vi "output.vi"(8 "error in":errorcluster, 10 "data table in":T1, 11 "SystemLin Tag Module runtime in":refnum<class "SystemLink File runtime.lvclass">) -> (0 "error out":errorcluster, 2 "data table out":T1, 3 "SystemLin Tag Module runtime out":refnum<class "SystemLink File runtime.lvclass">)   [LabVIEW 2015, in "SystemLink File runtime.lvclass"]
doc: "Provides an interface for writing data to a module at runtime. While this interface performs no operations, a child should provide an override which may write to any open sessions, references, or interfaces."
uses:
  SystemLink File runtime.lvclass
  <vilib>/NI/Tag Bus/table/data table.ctl
  SystemLink File runtime.lvclass/SystemLink File runtime.ctl
  <vilib>/NI/Tag Bus/table/data polymorphs/read one/read Boolean.vi
  <vilib>/Skyline/File/File/Send File.vi
  <vilib>/NI/Tag Bus/table/data table.lvlib
  <vilib>/NI/Tag Bus/table/data polymorphs/read one/read Double.vi
  <vilib>/NI/Tag Bus/table/data polymorphs/read one/read Single.vi
  <vilib>/NI/Tag Bus/table/data polymorphs/read one/read I32.vi
  <vilib>/NI/Tag Bus/table/data polymorphs/read one/read I16.vi
  <vilib>/NI/Tag Bus/table/data polymorphs/read one/read I8.vi
  <vilib>/Skyline/Tag/Wrapper/Wrapper_class/NI Skyline Tag.lvclass
  <vilib>/Skyline/Tag/Wrapper/Wrapper_class/Write Tag (DBL).vi
  <vilib>/Skyline/Tag/Wrapper/Wrapper_class/Write Tag (I32).vi
  <vilib>/NI/Tag Bus/table/data polymorphs/read one/read String.vi
  <vilib>/Skyline/Tag/Wrapper/Wrapper_class/Write Tag (String).vi
  <vilib>/Skyline/File/File/NI Skyline File.lvclass
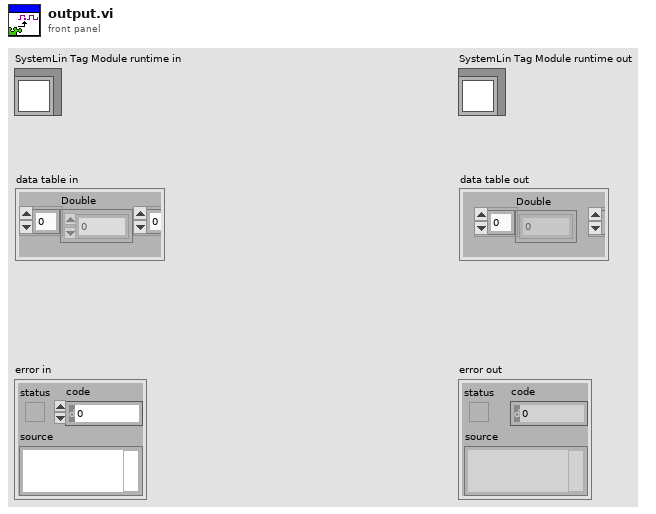
[diagram p1: front panel]
types:
  T1 = typedef "tag bus.lvlib/data table.lvlib/data table.ctl" = cluster{"Double":dbl[], "Single":sgl[], "I64":i64[], "I32":i32[], "I16":i16[], "I8":i8[], "U64":u64[], "U32":u32[], "U16":u16[], "U8":u8[], "Boolean":bool[], "String":string[], "Array of Double":cluster{"DBL Array":dbl[]}[], "Array of Single":cluster{"SGL Array":sgl[]}[], "Array of I64":cluster{"I64 Array":i64[]}[], "Array of I32":cluster{"I32 Array":i32[]}[], "Array of I16":cluster{"I16 Array":i16[]}[], "Array of I8":cluster{"I8 Array":i8[]}[], "Array of U64":cluster{"U64 Array":u64[]}[], "Array of U32":cluster{"U32 Array":u32[]}[], "Array of U16":cluster{"U16 Array":u16[]}[], "Array of U8":cluster{"U8 Array":u8[]}[], "Array of Boolean":cluster{"Boolean Array":bool[]}[], "Array of String":cluster{"String Array":string[]}[]}
  T2 = typedef "SystemLink File configuration.lvclass/SysLink Mapping.ctl" = cluster{"Data Type":T3, "Tag Reference":refnum<class "NI Skyline Tag.lvclass">, "Tag Bus Index":i32, "AMQP":bool, "Skylink Index":i32}
  T3 = typedef "SystemLink File configuration.lvclass/Data Tag Type.ctl" = enum16{"Double", "Single", "I32", "I16", "I8", "U64", "U32", "U16", "U8", "Boolean", "String", "Timestamp"}
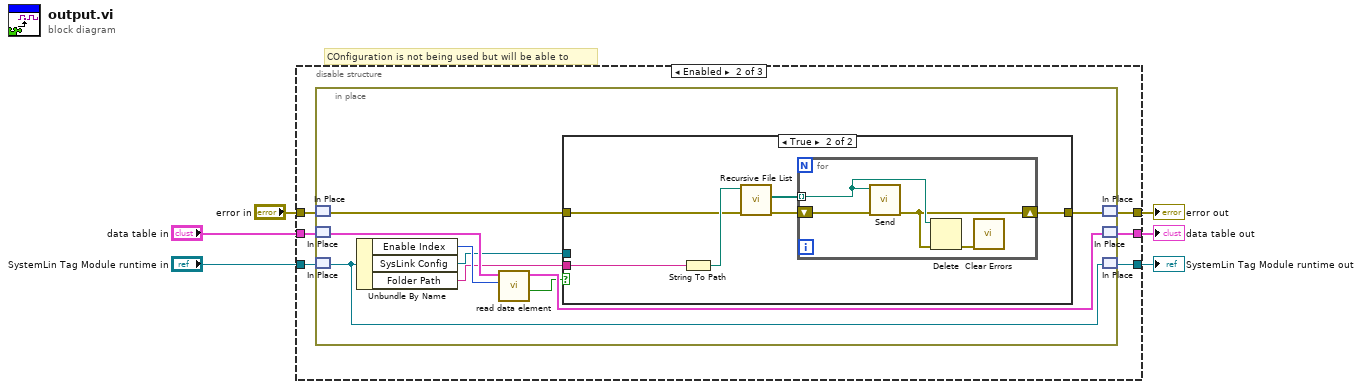
[diagram p0: block diagram]
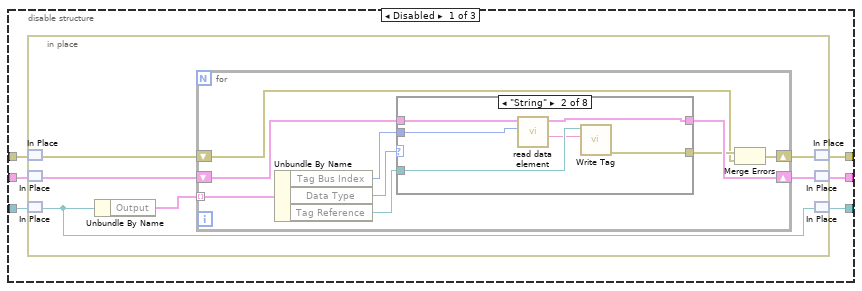
[diagram p2: hidden frame]
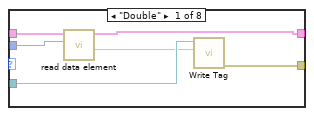
[diagram p3: hidden frame]
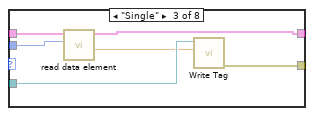
[diagram p4: hidden frame]
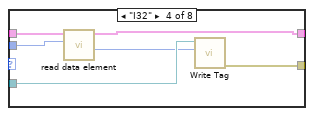
[diagram p5: hidden frame]
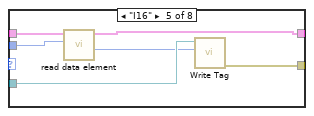
[diagram p6: hidden frame]
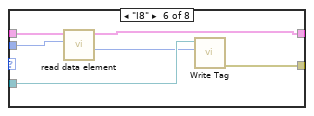
[diagram p7: hidden frame]
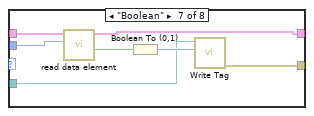
[diagram p8: hidden frame]
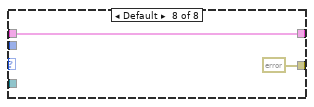
[diagram p9: hidden frame]
diagram:
  # "COnfiguration is not being used but will be able to"
  n1 = disable-structure shown="Enabled" {
    disable-tunnel: "SystemLin Tag Module runtime in" -> [w12 w78 _]
    disable-tunnel: [w11 w77 _] -> w5
    disable-tunnel: [w10 w76 _] -> w4
    disable-tunnel: [w9 w75 _] -> w3
    disable-tunnel: "data table in" -> [w8 w74 _]
    disable-tunnel: "error in" -> [w7 w73 _]
    frame Disabled {
      n2 = in-place {
        n3 = in-place-match #1(w7) -> (w14:errorcluster)
        n4 = in-place-match #2(w8) -> (w18:T1)
        n5 = in-place-match #3(w12) -> (w16:refnum<class "SystemLink File runtime.lvclass">)
        n6 = Unbundle By Name(w16) -> ("Output"=w15:T2[])
        n7 = for {
          shift-right: [w24] -> w17
          shift-left: w18 -> [w25]
          tunnel: w15 -> [w27] mode=indexing
          shift-right: [w19] -> w13
          shift-left: w14 -> [w20]
          n8 = Unbundle By Name(w27) -> ("Tag Bus Index"=w22:i32, "Data Type"=w26:T3, "Tag Reference"=w23:refnum<class "NI Skyline Tag.lvclass">)
          n9 = case shown="\"String\"" w26 {
            tunnel: w25 -> [w33 w39 w45 w51 w57 w63 w70 w72]
            tunnel: [w31 w37 w43 w49 w55 w61 w68 w72] -> w24
            tunnel: w23 -> [w30 w36 w42 w48 w54 w60 w64 _]
            tunnel: [w28 w34 w40 w46 w52 w58 w67 errorcluster {"status"=FALSE, "code"=0, "source"=""} ("error IO")] -> w21
            tunnel: w22 -> [w32 w38 w44 w50 w56 w62 w69 _]
            frame "Double" {
              n10 = call-poly <vilib>:"read data element.vi"("index"=w32, "data table in"=w33) -> ("value"=w29:dbl, "data table out"=w31:T1)  [unwired: 8 in]
              n11 = call-poly <vilib>:"Write Tag.vi"("value"=w29, "tag in"=w30) -> ("error out"=w28:errorcluster)  [unwired: 8 in, 1 out]
            }
            frame "String" {
              n12 = call-poly <vilib>:"read data element.vi"("index"=w38, "data table in"=w39) -> ("value"=w35:string, "data table out"=w37:T1)  [unwired: 8 in]
              n13 = call-poly <vilib>:"Write Tag.vi"("value"=w35, "tag in"=w36) -> ("error out"=w34:errorcluster)  [unwired: 8 in, 1 out]
            }
            frame "Single" {
              n14 = call-poly <vilib>:"read data element.vi"("index"=w44, "data table in"=w45) -> ("value"=w41:sgl, "data table out"=w43:T1)  [unwired: 8 in]
              n15 = call-poly <vilib>:"Write Tag.vi"("value"=w41, "tag in"=w42) -> ("error out"=w40:errorcluster)  [unwired: 8 in, 1 out]
            }
            frame "I32" {
              n16 = call-poly <vilib>:"read data element.vi"("index"=w50, "data table in"=w51) -> ("value"=w47:i32, "data table out"=w49:T1)  [unwired: 8 in]
              n17 = call-poly <vilib>:"Write Tag.vi"("value"=w47, "tag in"=w48) -> ("error out"=w46:errorcluster)  [unwired: 8 in, 1 out]
            }
            frame "I16" {
              n18 = call-poly <vilib>:"read data element.vi"("index"=w56, "data table in"=w57) -> ("value"=w53:i16, "data table out"=w55:T1)  [unwired: 8 in]
              n19 = call-poly <vilib>:"Write Tag.vi"("value"=w53, "tag in"=w54) -> ("error out"=w52:errorcluster)  [unwired: 8 in, 1 out]
            }
            frame "I8" {
              n20 = call-poly <vilib>:"read data element.vi"("index"=w62, "data table in"=w63) -> ("value"=w59:i8, "data table out"=w61:T1)  [unwired: 8 in]
              n21 = call-poly <vilib>:"Write Tag.vi"("value"=w59, "tag in"=w60) -> ("error out"=w58:errorcluster)  [unwired: 8 in, 1 out]
            }
            frame "Boolean" {
              n22 = call-poly <vilib>:"read data element.vi"("index"=w69, "data table in"=w70) -> ("value"=w65:bool, "data table out"=w68:T1)  [unwired: 8 in]
              n23 = Boolean To (0,1)(Boolean=w65) -> (0, 1=w66:i16)
              n24 = call-poly <vilib>:"Write Tag.vi"("value"=w66, "tag in"=w64) -> ("error out"=w67:errorcluster)  [unwired: 8 in, 1 out]
            }
            frame Default {
            }
          }
          n25 = Merge Errors(w21, w20) -> (w19:errorcluster)
        }
        n26 = in-place-match #1(w13) -> (w9:errorcluster)
        n27 = in-place-match #2(w17) -> (w10:T1)
        n28 = in-place-match #3(w16) -> (w11:refnum<class "SystemLink File runtime.lvclass">)
      }
    }
    frame Enabled {
      n29 = in-place {
        n30 = in-place-match #4(w73) -> (w81:errorcluster)
        n31 = in-place-match #5(w74) -> (w86:T1)
        n32 = in-place-match #6(w78) -> (w87:refnum<class "SystemLink File runtime.lvclass">)
        n33 = Unbundle By Name(w87) -> ("Enable Index"=w84:i32, "SysLink Config"=w82:refnum<class "NI Skyline Configuration.lvclass">, "Folder Path"=w79:string)
        n34 = call-poly <vilib>:"read data element.vi"("index"=w84, "data table in"=w86) -> ("value"=w83:bool, "data table out"=w85:T1)  [unwired: 8 in]
        n35 = case shown="True" w83 {
          tunnel: w82 -> [_ _]
          tunnel: w81 -> [w88 w91]
          tunnel: [w88 w94] -> w80
          tunnel: w79 -> [_ w92]
          frame False {
          }
          frame True {
            n36 = String To Path(string=w92) -> (path=w93:path)
            n37 = call <vilib>:"Recursive File List.vi"("error in (no error)"=w91, "Folder Path"=w93) -> ("error out"=w90:errorcluster, "All Files in Dir"=w89:path[])  [unwired: 5 in, 3 out]
            n38 = for {
              shift-right: [w95] -> w94
              shift-left: w90 -> [w98]
              tunnel: w89 -> [w97] mode=indexing
              n39 = call-poly <vilib>:"Send.vi"("error in (no error)"=w98, "path"=w97) -> ("error out"=w95:errorcluster)  [unwired: 7 in, 1 out]
              n40 = Delete(path (use dialog)=w97, error in=w95) -> (error out=w96:errorcluster)  [unwired: 3 in, 2 out]
              n41 = call <vilib>:"Clear Errors.vi"("error in (no error)"=w96) -> ()  [unwired: 5 in, 2 out]
            }
          }
        }
        n42 = in-place-match #4(w80) -> (w75:errorcluster)
        n43 = in-place-match #5(w85) -> (w76:T1)
        n44 = in-place-match #6(w87) -> (w77:refnum<class "SystemLink File runtime.lvclass">)
      }
    }
    frame Disabled {
    }
  }
  "error out" <- w3
  "SystemLin Tag Module runtime out" <- w5
  "data table out" <- w4
